vi "full adder using half adder as sub vi.vi"() -> ()   [LabVIEW 2024]
panel:
  out "carry":bool
  out "Sum":bool
  in  "C":bool
  in  "B":bool
  in  "A":bool
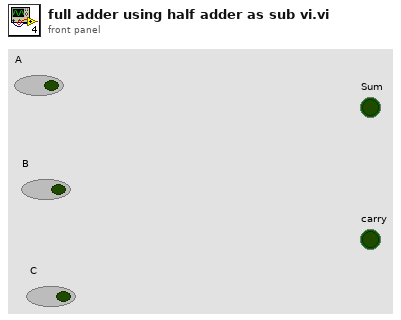
[diagram p1: front panel]
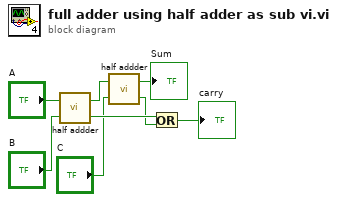
[diagram p0: block diagram]
diagram:
  n1 = call "half addder.vi"("b"="B", "a"="A") -> ("carry"=w4:bool, "sum"=w6:bool)
  n2 = call "half addder.vi"("b"="C", "a"=w6) -> ("carry"=w3:bool, "sum"=→"Sum":bool)
  n3 = Or(x=w4, y=w3) -> (x .or. y?=→"carry":bool)
